vi "Start Autobalancing.vi"(8 "error in (no error)":errorcluster, 9 "L2 Control":bool=TRUE caption="LBCB 2", 10 "L1 Control":bool=TRUE caption="LBCB 1", 11 "Number of\nLBCBs In":T1) -> (0 "error out":errorcluster, 1 "L2 Control Out":bool caption="LBCB 2", 2 "L1 Control Out":bool caption="LBCB 1")   [LabVIEW 2013]
uses:
  lib/Data Access Objects/Application/Number Of LBCBs.ctl
panel:
  in  "OK Button":bool
  # "WARNING: Autobalancing can destroy \nyour specimen!\nMake sure the oil pressure is off before starting."
  # "WARNING: LBCBs that are skipped cannot have oil pressure\napplied at anytime because the LBCB will jump to the zero\nposition."
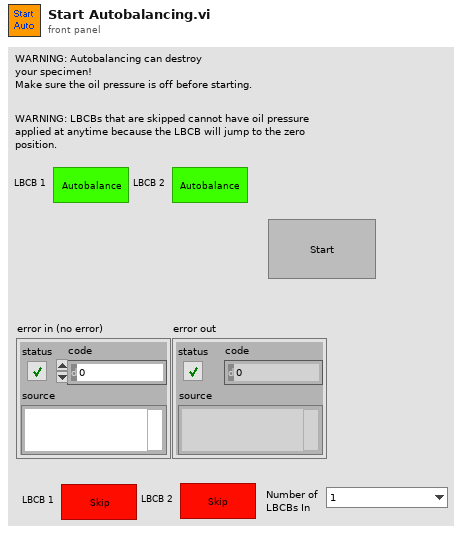
[diagram p1: front panel]
types:
  T1 = typedef "Number Of LBCBs.ctl" = enum16{"1", "2"}
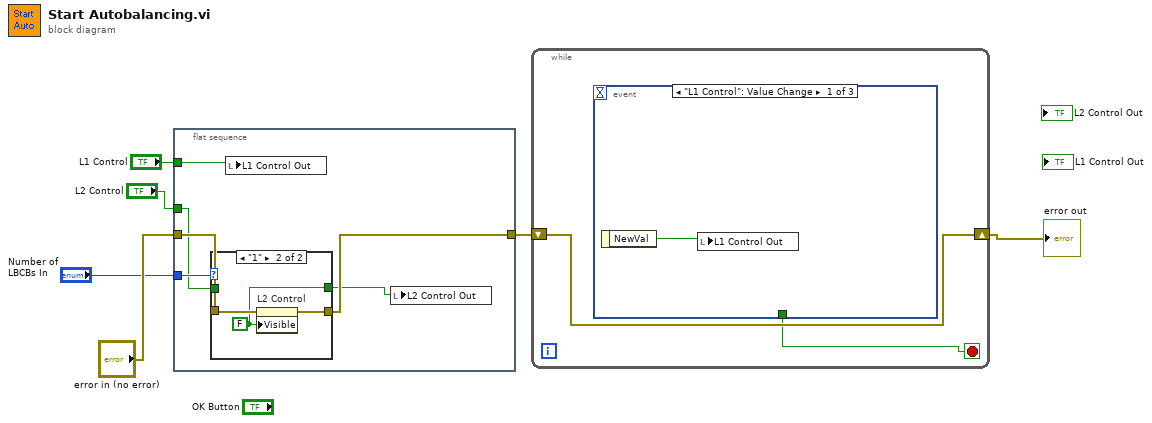
[diagram p0: block diagram]
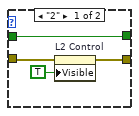
[diagram p2: hidden frame]
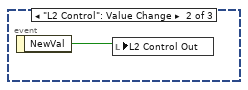
[diagram p3: hidden frame]
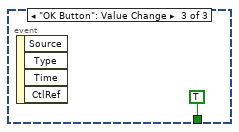
[diagram p4: hidden frame]
diagram:
  n1 = flat-sequence {
    tunnel: "L1 Control" -> [w12]
    tunnel: "L2 Control" -> [w8]
    tunnel: "error in (no error)" -> [w10]
    tunnel: [w9] -> w3
    tunnel: "Number of\nLBCBs In" -> [w11]
    frame #0 {
      n2 = case shown="\"1\"" w11 {
        tunnel: w10 -> [w15 w19]
        tunnel: [w14 w18] -> w9
        tunnel: w8 -> [w13 _]
        tunnel: [w13 w17] -> w7
        frame "2" {
          n3 = property on="L2 Control" class="Bool (strict)"(error in=w15, "Visible"=TRUE) -> (error out=w14:errorcluster)  [unwired: 1 in, 1 out]
        }
        frame "1" {
          w17 = FALSE ("Visible")
          n4 = property on="L2 Control" class="Bool (strict)"(error in=w19, "Visible"=w17) -> (error out=w18:errorcluster)  [unwired: 1 in, 1 out]
        }
      }
      n5 = local write "L1 Control Out"(w12) -> ()
      n6 = local write "L2 Control Out"(w7) -> ()
    }
  }
  n7 = while {
    shift-right: [w21] -> w2
    shift-left: w3 -> [w21]
    stop <- w20 stop-if-true
    n8 = event shown="[0] \"L1 Control\": Value Change" {
      selector: _ -> [_ _ _]
      dyn-events: _ -> [_ _ _]
      timeout: _ -> [_ _ _]
      tunnel: [_ _ TRUE] -> w20
      event "L1 Control": Value Change {
        n9 = event-data() -> ("NewVal"=w22:bool)  [unwired: 1 in]
        n10 = local write "L1 Control Out"(w22) -> ()
      }
      event "L2 Control": Value Change {
        n11 = event-data() -> ("NewVal"=w23:bool)  [unwired: 1 in]
        n12 = local write "L2 Control Out"(w23) -> ()
      }
      event "OK Button": Value Change {
        n13 = event-data() -> ()  [unwired: 1 in, 4 out]
      }
    }
  }
  "error out" <- w2
